vi "PlaneFit_flt.vi"(6 "Planing y/n?":bool, 7 "Reset Clicks":bool, 8 "Y PEN":dbl, 9 "Z":dbl, 10 "Nano Z":dbl, 11 "X":dbl) -> (2 "Plane Height (m)":dbl, 3 "Clicks":i32, 5 "Planing Done?":bool)   [LabVIEW 2019]
uses:
  GlobalClicksHeight_flt.vi
  <userlib>/HapticSTM/HapticSTM.lvlib
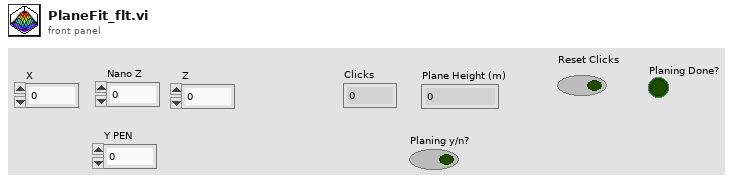
[diagram p1: front panel]
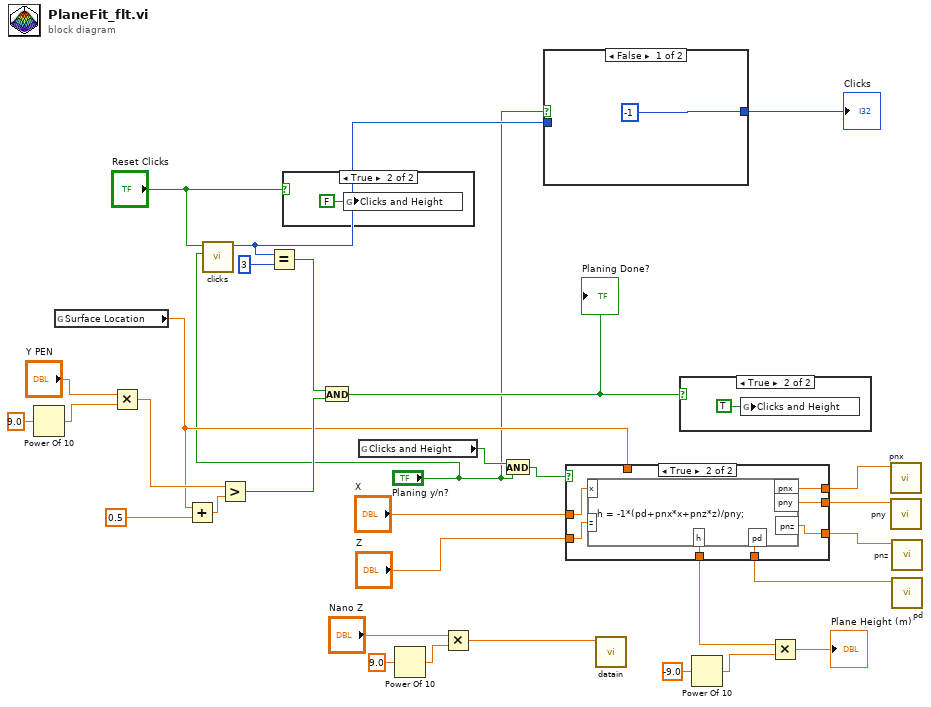
[diagram p0: block diagram]
diagram:
  n1 = Power Of 10(x=9.0) -> (10^x=w18:dbl)
  n2 = global read "GlobalClicksHeight_flt.vi" "Surface Location"() -> (w6:dbl)
  n3 = Multiply(x="Y PEN", y=w18) -> (x*y=w15:dbl)
  n4 = Add(x=w6, y=0.5) -> (x+y=w21:dbl)
  n5 = call <userlib>:"clicks.vi"("planing"="Planing y/n?", "reset"="Reset Clicks") -> ("function return"=w3:i32)  [unwired: 9 in]
  n6 = Greater?(x=w15, y=w21) -> (0:w22:bool)
  n7 = Equal?(x=w3, y=3) -> (x = y?=w23:bool)
  n8 = case shown="True" "Reset Clicks" {
    frame False {
    }
    frame True {
      n9 = global write "GlobalClicksHeight_flt.vi" "Clicks and Height"(FALSE ("Clicks and Height")) -> ()
    }
  }
  n10 = And(x=w23, y=w22) -> (x .and. y?=w19:bool)
  "Planing Done?" <- w19
  n11 = global read "GlobalClicksHeight_flt.vi" "Clicks and Height"() -> (w5:bool)
  n12 = Power Of 10(x=9.0) -> (10^x=w14:dbl)
  n13 = Multiply(x="Nano Z", y=w14) -> (x*y=w9:dbl)
  n14 = And(x=w5, y="Planing y/n?") -> (x .and. y?=w4:bool)
  n15 = case shown="False" "Planing y/n?" {
    tunnel: w3 -> [_ w34]
    tunnel: [-1 ("function return") w34] -> w2
    frame False {
    }
    frame True {
    }
  }
  "Clicks" <- w2
  n16 = call <userlib>:"datain.vi"("output"=w9) -> ()  [unwired: 11 in]
  n17 = case shown="True" w19 {
    frame False {
    }
    frame True {
      n18 = global write "GlobalClicksHeight_flt.vi" "Clicks and Height"(TRUE ("Clicks and Height")) -> ()
    }
  }
  n19 = Power Of 10(x=-9.0) -> (10^x=w26:dbl)
  n20 = call <userlib>:"pnx.vi"() -> ("function return"=w28:dbl)  [unwired: 11 in]
  n21 = call <userlib>:"pny.vi"() -> ("function return"=w27:dbl)  [unwired: 11 in]
  n22 = call <userlib>:"pnz.vi"() -> ("function return"=w31:dbl)  [unwired: 11 in]
  n23 = call <userlib>:"pd.vi"() -> ("function return"=w30:dbl)  [unwired: 11 in]
  n24 = case shown="True" w4 {
    tunnel: "X" -> [_ w43]
    tunnel: w28 -> [_ w41]
    tunnel: w27 -> [_ w40]
    tunnel: w31 -> [_ w39]
    tunnel: w30 -> [_ w38]
    tunnel: "Z" -> [_ w42]
    tunnel: [w36 w37] -> w10
    tunnel: w6 -> [w36 _]
    frame False {
    }
    frame True {
      n25 = formula code="h = -1*(pd+pnx*x+pnz*z)/pny;"("x"=w43, "z"=w42, "pnx"=w41, "pnz"=w39, "pd"=w38, "pny"=w40) -> ("h"=w37:dbl)
    }
  }
  n26 = Multiply(x=w10, y=w26) -> (x*y=→"Plane Height (m)":dbl)
